vi "Load Test Image.vi"(8 "Error In":errorcluster) -> (0 "Error Out":errorcluster, 3 "Image":T1(plugin-control))   [LabVIEW 2018]
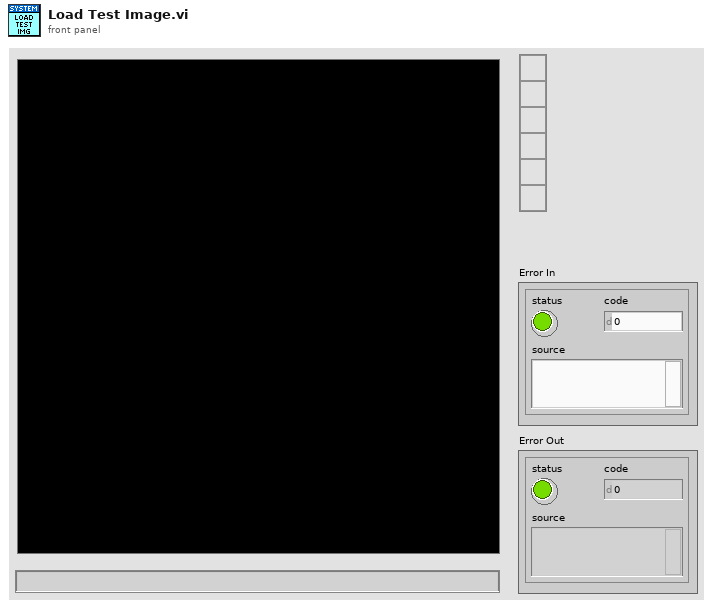
[diagram p1: front panel]
types:
  T1 = typedef "IMAQ Image.ctl" = refnum<image>
  T2 = cluster{"Read Raw File":i32, "File Data Type":u32, "Offset to Data":i32, "Use Min Max":enum32{"Don't use min max", "Use file values", "Use optional values"}, "Optional Min Value":sgl, "Optional Max Value":sgl, "Byte Order":enum32{"Big endian (Motorola)", "Little endian (Intel)"}}
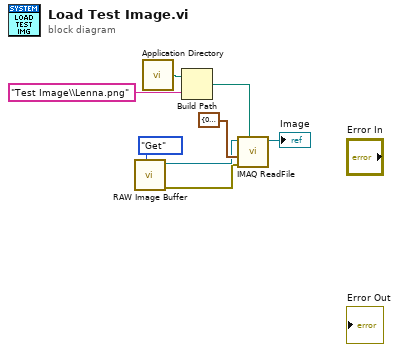
[diagram p0: block diagram]
diagram:
  n1 = call "RAW Image Buffer.vi"("Actions"=enum16{"Init", "Create", "Get", "Dispose"}."Get") -> ("Error Out"=w1:errorcluster, "Image Out"=w2:T1)  [unwired: 9 in]
  n2 = call <vilib>:"Application Directory.vi"() -> ("Application Directory"=w8:path)
  n3 = Build Path(base path=w8, name or relative path="Test Image\\Lenna.png") -> (appended path=w6:path)
  n4 = call "IMAQ ReadFile"("File Path"=w6, "error in (no error)"=w1, "File Options"=T2 {"Read Raw File"=0, "File Data Type"=5, "Offset to Data"=0, "Use Min Max"=enum."Don't use min max", "Optional Min Value"=0.0, "Optional Max Value"=0.0, "Byte Order"=enum."Big endian (Motorola)"}, "Image"=w2) -> ("Image Out"=→"Image":T1)  [unwired: 3 in, 4 out]
